vi "Tacho_and_Force_Calibration_MIKE2.vi"(9 "Force Ref In":T1, 10 "Tacho Ref In":T1, 11 "Calibration_Length":dbl) -> (2 "Force_calib_value":dbl, 3 "Velocity_calib_value":dbl)   [LabVIEW 2015]
uses:
  <vilib>/myRIO/Instrument Drivers/Onboard IO/AI/typedefs/AI Reference.ctl
  <vilib>/myRIO/Common/Instrument Driver Framework/Utilities/typedefs/myRIO Generic Hardware Reference.ctl
  <vilib>/myRIO/Common/Instrument Driver Framework/Utilities/typedefs/Hardware Version Enum.ctl
  <vilib>/myRIO/Common/Instrument Driver Framework/Utilities/typedefs/myRIO v1.0 Reference.ctl
  <vilib>/myRIO/Common/Instrument Driver Framework/Utilities/typedefs/Generic FPGA Reference.ctl
  <vilib>/myRIO/Common/Instrument Driver Framework/myRIO v1.0/AI/typedefs/AI Channels List.ctl
  <vilib>/myRIO/Common/Instrument Driver Framework/myRIO v1.0/AI/typedefs/AI Channels Enum.ctl
  <vilib>/myRIO/Common/Instrument Driver Framework/Utilities/typedefs/Analog Scaling Constants List.ctl
  <vilib>/myRIO/Common/Instrument Driver Framework/Utilities/typedefs/Analog Scaling Constants.ctl
  <vilib>/Utility/error.llb/Error Cluster From Error Code.vi
  <vilib>/myRIO/Common/Instrument Driver Framework/myRIO v1.0/AI/vis/myRIO v1.0 Read AI.vi
  <vilib>/myRIO/Instrument Drivers/Onboard IO/AI/AI.lvlib
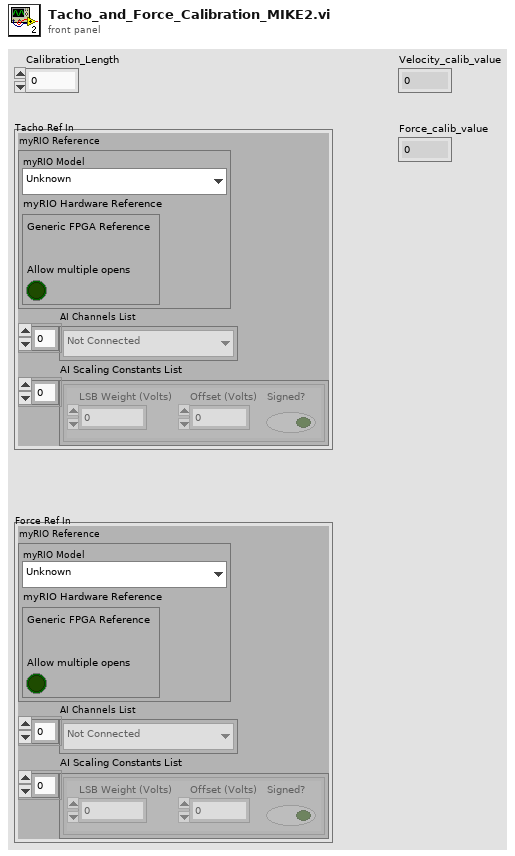
[diagram p1: front panel]
types:
  T1 = typedef "AI.lvlib/AI Reference.ctl" = cluster{"myRIO Reference":T2, "AI Channels List":T6, "AI Scaling Constants List":T8}
  T2 = typedef "myRIO Generic Hardware Reference.ctl" = cluster{"myRIO Model":T3, "myRIO Hardware Reference":T4}
  T3 = typedef "Hardware Version Enum.ctl" = enum16{"Unknown", "myRIO-1900", "myRIO-1950", "roboRIO"}
  T4 = typedef "myRIO v1.0 Reference.ctl" = cluster{"Generic FPGA Reference":T5, "Allow multiple opens":bool}
  T5 = typedef "Generic FPGA Reference.ctl" = refnum<k20>
  T6 = typedef "AI Channels List.ctl" = T7[]
  T7 = typedef "AI Channels Enum.ctl" = enum16{"Not Connected", "AudioIn/Left", "AudioIn/Right", "C/AI0", "C/AI1", "A/AI0", "A/AI1", "A/AI2", "A/AI3", "B/AI0", "B/AI1", "B/AI2", "B/AI3", "AI/AI0", "AI/AI1", "AI/AI2", "AI/AI3"}
  T8 = typedef "Analog Scaling Constants List.ctl" = T9[]
  T9 = typedef "Analog Scaling Constants.ctl" = cluster{"LSB Weight (Volts)":dbl, "Offset (Volts)":dbl, "Signed?":bool}
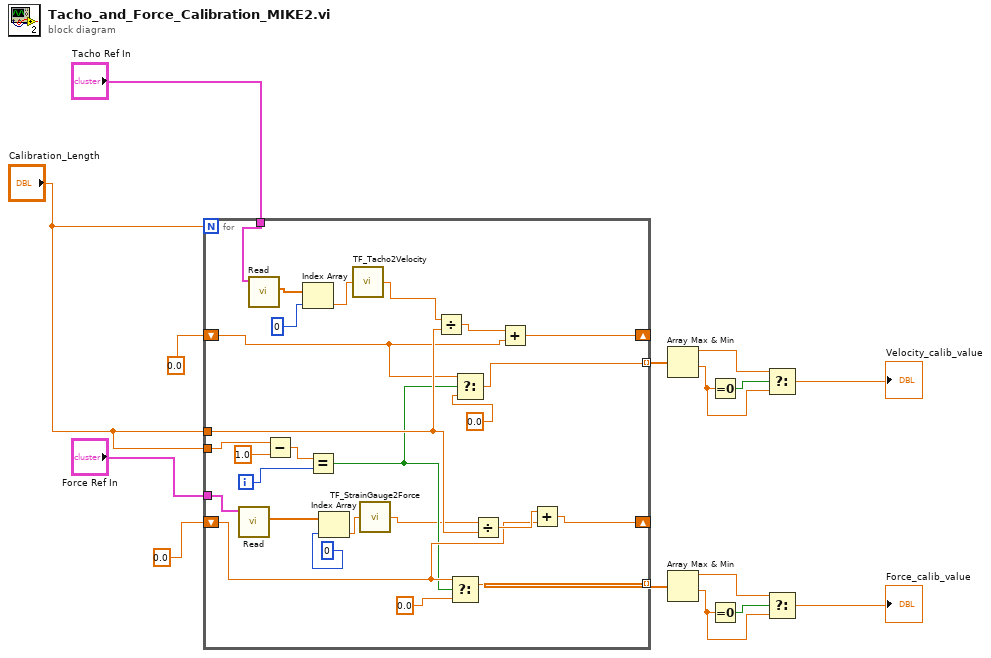
[diagram p0: block diagram]
diagram:
  n1 = for {
    N: "Calibration_Length" -> [_]
    tunnel: "Force Ref In" -> [w39]
    tunnel: "Calibration_Length" -> [w30]
    shift-right: [w37] -> _
    shift-left: 0.0 -> [w36]
    tunnel: "Calibration_Length" -> [w26]
    tunnel: [w34] -> w3 mode=indexing
    tunnel: "Tacho Ref In" -> [w31]
    shift-right: [w28] -> _
    shift-left: 0.0 -> [w23]
    tunnel: [w20] -> w14 mode=indexing
    i -> [w25]
    n2 = call <vilib>:"Read.vi"("AI Ref In"=w39) -> ("Values"=w40:dbl[])  [unwired: 8 in, 2 out]
    n3 = call <vilib>:"Read.vi"("AI Ref In"=w31) -> ("Values"=w33:dbl[])  [unwired: 8 in, 2 out]
    n4 = Subtract(x=w26, y=1.0) -> (x-y=w24:dbl)
    n5 = Index Array(array=w33, index=0) -> (element=w19:dbl)
    n6 = Equal?(x=w24, y=w25) -> (x = y?=w22:bool)
    n7 = Index Array(array=w40, index=0) -> (element=w17:dbl)
    n8 = call "TF_Tacho2Velocity.vi"("Motor Velocity Tacho Value [V]"=w19) -> ("Motor Velocity Tacho [deg/s]"=w18:dbl)  [unwired: 4 in]
    n9 = call "TF_StrainGauge2Force.vi"("Strain Gauge Value [V]"=w17) -> ("Force [N]"=w16:dbl)  [unwired: 4 in]
    n10 = Divide(x=w18, y=w30) -> (x/y=w29:dbl)
    n11 = Select(t=w36, s=w22, f=0.0) -> (s? t:f=w34:dbl)
    n12 = Select(t=w23, s=w22, f=0.0) -> (s? t:f=w20:dbl)
    n13 = Divide(x=w16, y=w30) -> (x/y=w38:dbl)
    n14 = Add(x=w29, y=w23) -> (x+y=w28:dbl)
    n15 = Add(x=w38, y=w36) -> (x+y=w37:dbl)
  }
  n16 = Array Max & Min(array=w14) -> (max value=w12:dbl, min value=w13:dbl)  [unwired: 2 out]
  n17 = Array Max & Min(array=w3) -> (max value=w6:dbl, min value=w7:dbl)  [unwired: 2 out]
  n18 = Equal To 0?(x=w13) -> (x = 0?=w11:bool)
  n19 = Equal To 0?(x=w7) -> (x = 0?=w5:bool)
  n20 = Select(t=w12, s=w11, f=w13) -> (s? t:f=→"Velocity_calib_value":dbl)
  n21 = Select(t=w6, s=w5, f=w7) -> (s? t:f=→"Force_calib_value":dbl)
